vi "connect tls client.vi"(8 "error in":errorcluster, 10 "servername":string, 11 "client":u64) -> (0 "error out":errorcluster, 3 "lvsocket":u64)   [LabVIEW 2016, in "lv tls dll.lvlib"]
uses:
  lv tls dll.lvlib
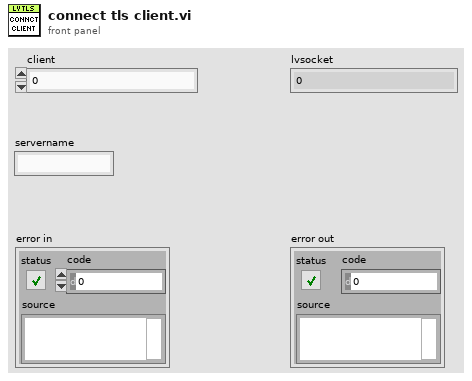
[diagram p1: front panel]
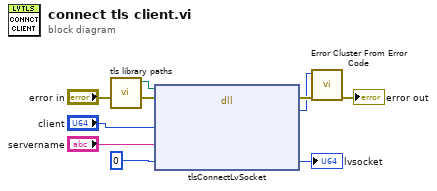
[diagram p0: block diagram]
diagram:
  n1 = call "tls library paths.vi"() -> ("lvtls"=w7:path)  [unwired: 8 in, 3 out]
  n2 = dll-call lib="C:/Users/IEUser/Desktop/tlssimple/lvlibtls.dll" fn="tlsConnectLvSocket"(path in=w7, error in="error in", "context"="client", "servername"="servername", "lvsocket"=u64 0) -> (error out=w9:errorcluster, "err"=w8:i32, "lvsocket"=→"lvsocket":u64)  [unwired: 3 in, 1 out]
  n3 = call <vilib>:"Error Cluster From Error Code.vi"("error in (no error)"=w9, "error code (0)"=w8) -> ("error out"=→"error out":errorcluster)  [unwired: 7 in]
